vi "OAT Even Angle Signal Subset.vi"   [LabVIEW 2017, in "SoundVib_OAUtility.lvlib"]
doc: "Retrieves a subset of an even-angle signal at a specified revolution duration. This VI does not maintain state internally; you can use this VI in a loop to process multiple blocks. Wire data to the <B>even-angle signal</B> input to determine the polymorphic instance to use or manually select the instance."
uses:
  <vilib>/addons/Sound and Vibration/Order Analysis/Utility/SoundVib_OAUtility.lvlib
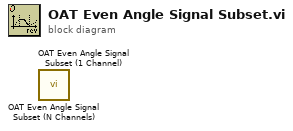
[diagram p0: block diagram]
diagram:
  n1 = call <vilib>:"OAT Even Angle Signal Subset (N Channels).vi"() -> ()  [unwired: 13 in, 3 out]
  n2 = call <vilib>:"OAT Even Angle Signal Subset (1 Channel).vi"() -> ()  [unwired: 13 in, 3 out]
